vi "Write Command Status.vi"(8 "error in (no error)":errorcluster, 10 "Command Status":T1, 11 "Command Processor in":refnum<class "Command Processor.lvclass">) -> (0 "error out":errorcluster, 3 "Command Processor out":refnum<class "Command Processor.lvclass">)   [LabVIEW 2013, in "Command Processor.lvlib" / "Command Processor.lvclass"]
uses:
  Command Processor.lvclass
  Command/Command Status.ctl
  Command/State Status.ctl
  Command Processor.lvclass/Command Processor.ctl
  <vilib>/ActorFramework/Actor/Actor.lvclass
  Command/Command.lvclass
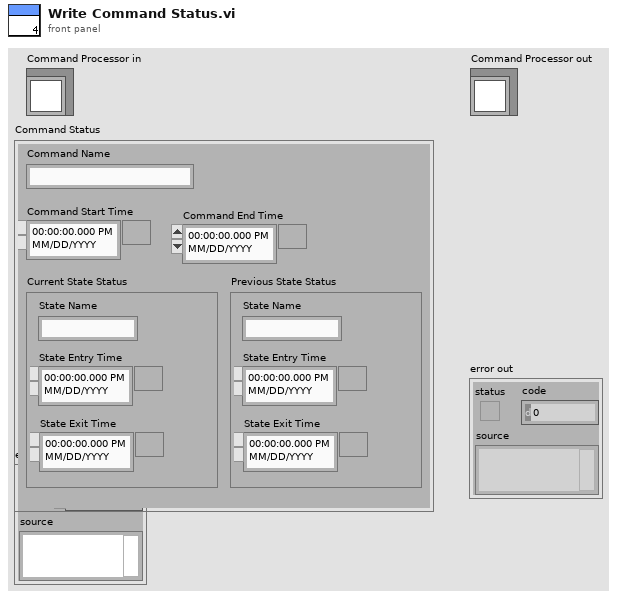
[diagram p1: front panel]
types:
  T1 = typedef "Command Processor.lvlib/Command.lvlib/Command.lvclass/Command Status.ctl" = cluster{"Command Name":string, "Current State Status":T2, "Command Start Time":timestamp, "Command End Time":timestamp, "Previous State Status":T2}
  T2 = typedef "Command Processor.lvlib/Command.lvlib/Command.lvclass/State Status.ctl" = cluster{"State Name":string, "State Entry Time":timestamp, "State Exit Time":timestamp}
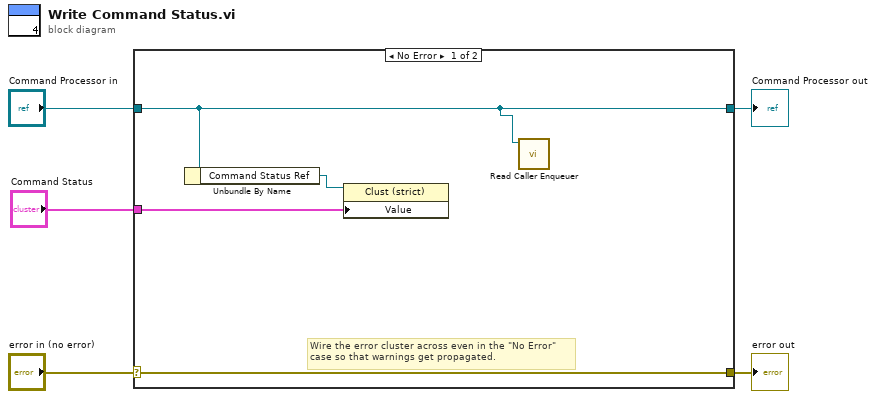
[diagram p0: block diagram]
diagram:
  n1 = case shown="No Error" "error in (no error)" {
    selector: "error in (no error)" -> [w9 w11]
    tunnel: [w9 w11] -> w4
    tunnel: [w6 w10] -> w2
    tunnel: "Command Processor in" -> [w6 w10]
    tunnel: "Command Status" -> [w7 _]
    frame No Error {
      # "Wire the error cluster across even in the \"No Error\"\ncase so that warnings get propagated."
      n2 = Unbundle By Name(w6) -> ("Command Status Ref"=w8:refnum<vi>)
      n3 = property class="Clust (strict)"(reference=w8, "Value"=w7) -> ()  [unwired: 1 in, 2 out]
      n4 = call <vilib>:"Read Caller Enqueuer.vi"("Actor"=w6) -> ()  [unwired: 10 in, 1 out]
    }
    frame Error {
    }
  }
  "error out" <- w4
  "Command Processor out" <- w2
